vi "Query Configuration Data.vi"(8 "error in (no error)":errorcluster, 11 "Ethernet in":refnum<class "ENET_BS120x.lvclass">) -> (0 "error out":errorcluster, 1 "Received":bool, 2 "Configuration Data":string, 3 "Ethernet out":refnum<class "ENET_BS120x.lvclass">)   [LabVIEW 2021, in "BS120x Driver.lvlib" / "ENET_BS120x.lvclass"]
uses:
  ENET_BS120x.lvclass
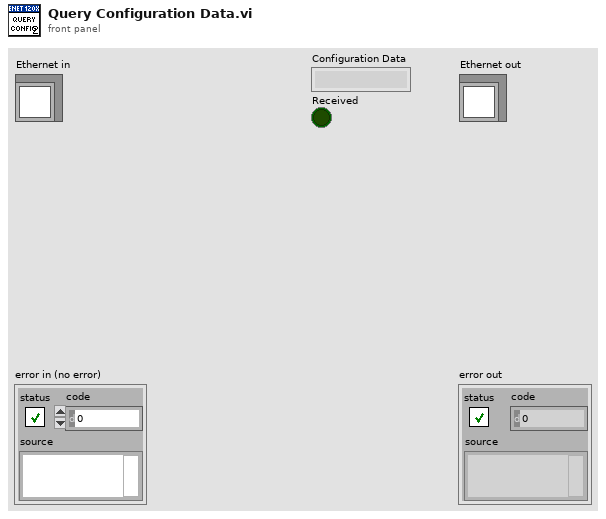
[diagram p1: front panel]
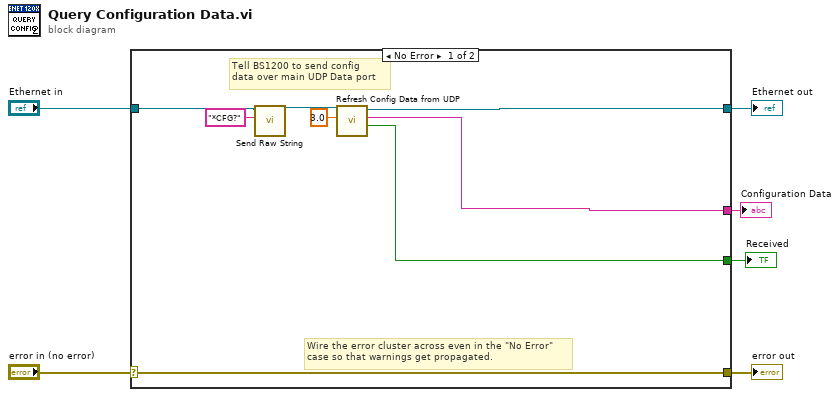
[diagram p0: block diagram]
diagram:
  n1 = case shown="No Error" "error in (no error)" {
    selector: "error in (no error)" -> [w14 w16]
    tunnel: [w14 w16] -> w5
    tunnel: [w12 w15] -> w3
    tunnel: "Ethernet in" -> [w9 w15]
    tunnel: [w11 _] -> w2
    tunnel: [w10 _] -> w1
    frame No Error {
      # "Tell BS1200 to send config\ndata over main UDP Data port"
      # "Wire the error cluster across even in the \"No Error\"\ncase so that warnings get propagated."
      n2 = call "Send Raw String.vi"("String Data"="*CFG?", "ENET in"=w9) -> ("ENET out"=w7:refnum<class "ENET_BS120x.lvclass">)  [unwired: 8 in, 1 out]
      n3 = call "Refresh Config Data from UDP.vi"("Timeout (2s)"=3.0, "Ethernet in"=w7) -> ("Received"=w10:bool, "Configuration Data"=w11:string, "Ethernet out"=w12:refnum<class "ENET_BS120x.lvclass">)  [unwired: 6 in, 1 out]
    }
    frame Error {
    }
  }
  "error out" <- w5
  "Ethernet out" <- w3
  "Configuration Data" <- w2
  "Received" <- w1
